vi "field timeout.vi"() -> ()   [LabVIEW 2021]
panel:
  out "Sweep Chart":dbl(graph)
  in  "timer on":bool
  in  "timer":dbl format="%.2f"
  in  "te":bool
  out "Clock":string="1:28:18 AM"
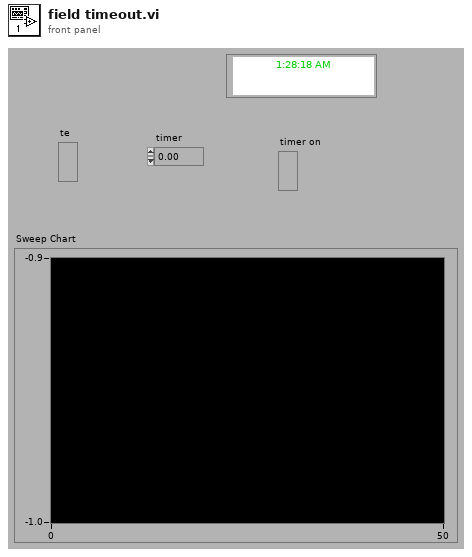
[diagram p1: front panel]
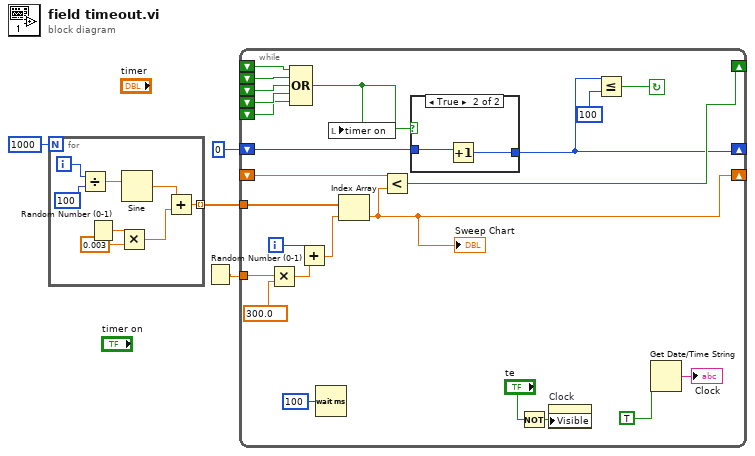
[diagram p0: block diagram]
diagram:
  n1 = for {
    N: 1000 -> [_]
    tunnel: [w5] -> w3 mode=indexing
    i -> [w12]
    n2 = Divide(x=w12, y=100) -> (x/y=w10:dbl)
    n3 = Random Number (0-1)() -> (number: 0 to 1=w8:dbl)
    n4 = Multiply(x=w8, y=0.003) -> (x*y=w6:dbl)
    n5 = Sine(x=w10) -> (sin(x)=w7:dbl)
    n6 = Add(x=w7, y=w6) -> (x+y=w5:dbl)
  }
  n7 = Random Number (0-1)() -> (number: 0 to 1=w2:dbl)
  n8 = while {
    shift-left: 0 -> [w14]
    shift-right: [w13] -> _
    shift-left: _ -> [w21]
    shift-left: _ -> [w22]
    shift-left: _ -> [w23]
    shift-left: _ -> [w24]
    shift-left: _ -> [w25]
    shift-right: [w26] -> _
    shift-left: _ -> [w27]
    shift-right: [w20] -> _
    tunnel: w2 -> [w32]
    tunnel: w3 -> [w29]
    i -> [w31]
    stop <- w15 continue-if-true
    n9 = Multiply(x=w32, y=300.0) -> (x*y=w30:dbl)
    n10 = Compound Arithmetic op=OR(w25, w24, w23, w22, w21) -> (w18:bool)
    n11 = Add(x=w31, y=w30) -> (x+y=w28:dbl)
    n12 = Wait (ms)(milliseconds to wait=u32 100) -> ()  [unwired: 1 out]
    n13 = local write "timer on"(w18) -> ()
    n14 = Index Array(array=w29, index=w28) -> (element=w20:dbl)
    "Sweep Chart" <- w20
    n15 = Less?(x=w27, y=w20) -> (x < y?=w26:bool)
    n16 = case shown="True" w18 {
      tunnel: [w37 w39] -> w13
      tunnel: w14 -> [w37 w38]
      frame False {
      }
      frame True {
        n17 = Increment(x=w38) -> (x+1=w39:i32)
      }
    }
    n18 = Not(x="te") -> (.not. x?=w35:bool)
    n19 = property on="Clock" class="Str"("Visible"=w35) -> ()  [unwired: 2 in, 2 out]
    n20 = Less Or Equal?(x=w13, y=100) -> (x <= y?=w15:bool)
    n21 = Get Date/Time String(want seconds? (F)=TRUE) -> (time string=→"Clock":string)  [unwired: 2 in, 1 out]
  }
